vi "Build Write Msg.vi"(0 "Siemens Ctr in":T1, 1 "Bit/Byte":u8(ring)=2 items=["Boolen"=1, "Byte"=2], 5 "#DB No.":u16, 7 "#offset":u32, 9 "Input":u8[](array[numeric]), 11 "error in (no error)":errorcluster, 12 "Address Areas":T2=132 items=["Input(I)"=129, "Output(Q)"=130, "Bit Memory(M)"=131, "Data(DB)"=132], 13 "#items":u16) -> (4 "Siemens Ctr out":T1, 6 "appended array":u8[](array[numeric]) format="%02x", 15 "error out":errorcluster)   [LabVIEW 2014, in "Simatic S7.lvlib"]
uses:
  Simatic S7.lvlib
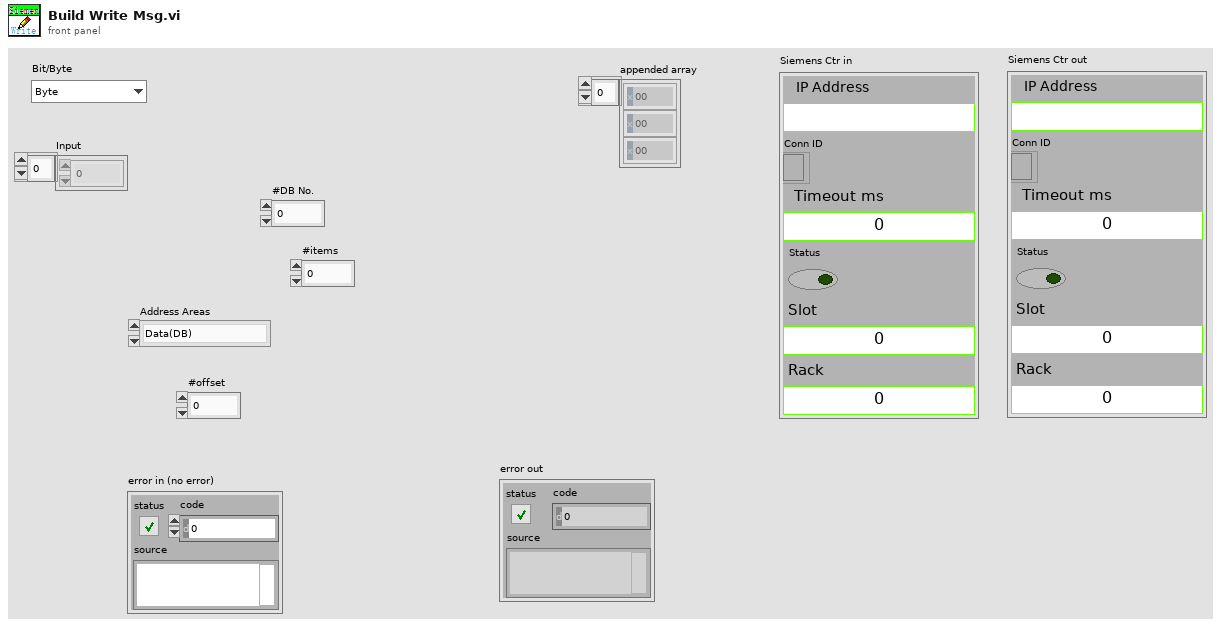
[diagram p1: front panel]
types:
  T1 = typedef "Simatic S7.lvlib/Siemens Ref.ctl" = cluster{"IP Address ":string, "Conn ID":refnum<k5>, "Timeout ms":i32, "Status":bool, "Slot":u16, "Rack":u16}
  T2 = typedef "Simatic S7.lvlib/Address Areas.ctl" = u8
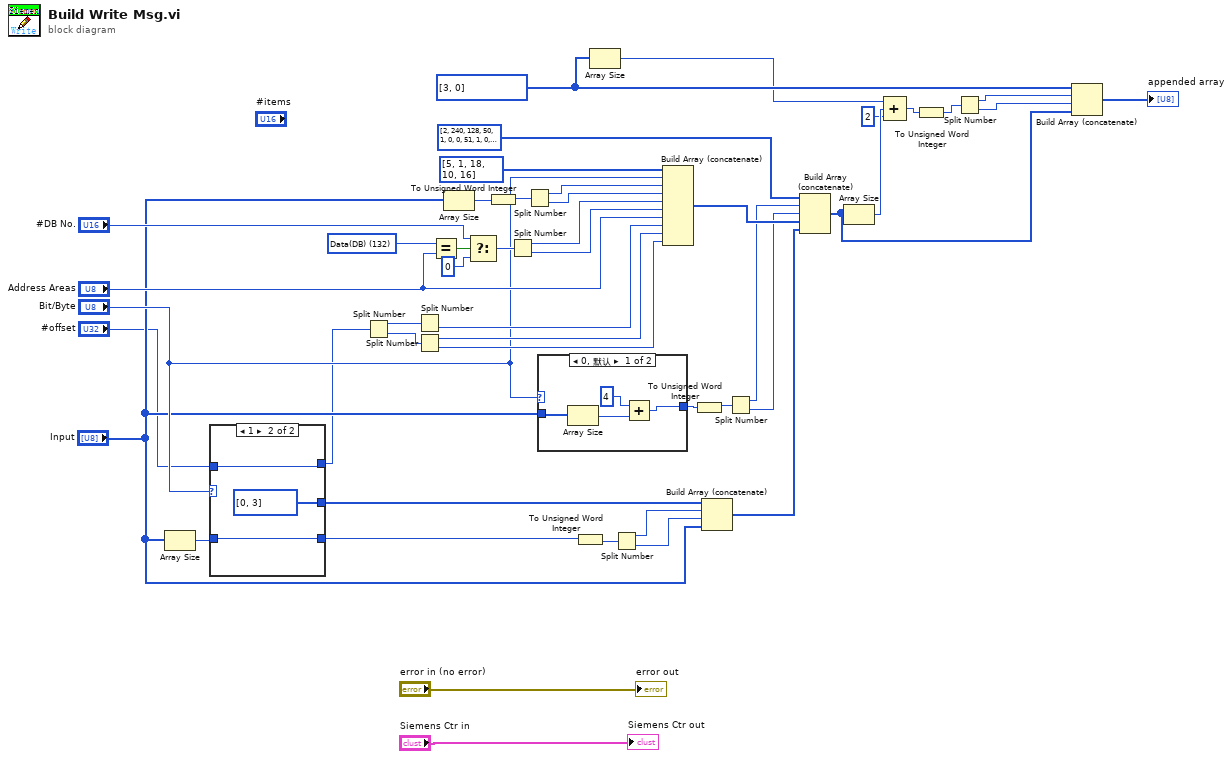
[diagram p0: block diagram]
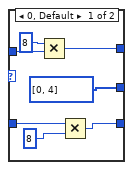
[diagram p2: hidden frame]
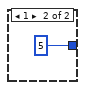
[diagram p3: hidden frame]
diagram:
  w31 = T2 132 items=["Input(I)"=129, "Output(Q)"=130, "Bit Memory(M)"=131, "Data(DB)"=132] ("Address Areas")
  w47 = u8[] [3, 0]
  n1 = Array Size(array="Input") -> (size(s)=w19:i32)
  n2 = case shown="1" "Bit/Byte" {
    tunnel: [u8[] [0, 4] u8[] [0, 3]] -> w16
    tunnel: w19 -> [w53 w56]
    tunnel: [w51 w56] -> w18
    tunnel: "#offset" -> [w50 w55]
    tunnel: [w48 w55] -> w1
    frame 0, Default {
      n3 = Multiply(x=u32 8, y=w50) -> (x*y=w48:u32)
      n4 = Multiply(x=w53, y=u8 8) -> (x*y=w51:i32)
    }
    frame 1 {
    }
  }
  n5 = Split Number(x=w1) -> (hi(x)=w25:u16, lo(x)=w24:u16)
  n6 = Split Number(x=w25) -> (lo(x)=w23:u8)  [unwired: 1 out]
  n7 = Split Number(x=w24) -> (hi(x)=w22:u8, lo(x)=w21:u8)
  n8 = Equal?(x=w31, y="Address Areas") -> (x = y?=w33:bool)
  n9 = Array Size(array="Input") -> (size(s)=w37:i32)
  n10 = Select(t="#DB No.", s=w33, f=u16 0) -> (s? t:f=w29:u16)
  n11 = To Unsigned Word Integer(number=w37) -> (unsigned 16bit integer=w36:u16)
  n12 = Split Number(x=w29) -> (hi(x)=w28:u8, lo(x)=w27:u8)
  n13 = Split Number(x=w36) -> (hi(x)=w35:u8, lo(x)=w34:u8)
  n14 = case shown="0, 默认" "Bit/Byte" {
    tunnel: "Input" -> [w61 _]
    tunnel: [w58 5 ("size(s)")] -> w40
    frame 0, Default {
      n15 = Array Size(array=w61) -> (size(s)=w60:i32)
      n16 = Add(x=4, y=w60) -> (x+y=w58:i32)
    }
    frame 1 {
    }
  }
  n17 = To Unsigned Word Integer(number=w18) -> (unsigned 16bit integer=w17:u16)
  n18 = Array Size(array=w47) -> (size(s)=w46:i32)
  n19 = Split Number(x=w17) -> (hi(x)=w15:u8, lo(x)=w14:u8)
  n20 = Build Array (concatenate)(u8[] [5, 1, 18, 10, 16], "Bit/Byte", w35, w34, w28, w27, "Address Areas", w23, w22, w21) -> (w12:T2[])
  n21 = To Unsigned Word Integer(number=w40) -> (unsigned 16bit integer=w39:u16)
  n22 = Build Array (concatenate)(w16, w15, w14, "Input") -> (w7:u8[])
  n23 = Split Number(x=w39) -> (hi(x)=w6:u8, lo(x)=w5:u8)
  n24 = Build Array (concatenate)(u8[] [2, 240, 128, 50, 1, 0, 0, 51, 1, 0, 14], w6, w5, w12, w7) -> (w10:T2[])
  n25 = Array Size(array=w10) -> (size(s)=w41:i32)
  n26 = Compound Arithmetic op=ADD(w46, w41, 2 ("value")) -> (w45:i32)
  n27 = To Unsigned Word Integer(number=w45) -> (unsigned 16bit integer=w44:u16)
  n28 = Split Number(x=w44) -> (hi(x)=w43:u8, lo(x)=w42:u8)
  n29 = Build Array (concatenate)(w47, w43, w42, w10) -> (→"appended array":T2[])
  "error out" <- "error in (no error)"
  "Siemens Ctr out" <- "Siemens Ctr in"
